vi "Relative Coordinates.vi"(1 "All Coordinates":cluster{"X":dbl, "Y":dbl}[](array[cluster]), 2 "Command Coordinates":cluster{"X":dbl, "Y":dbl}[](array[cluster])) -> (0 "Adjusted Command Coordinates":cluster{"X":dbl, "Y":dbl}[](array[cluster]))   [LabVIEW 2019]
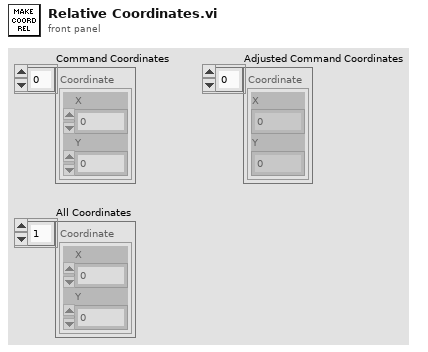
[diagram p1: front panel]
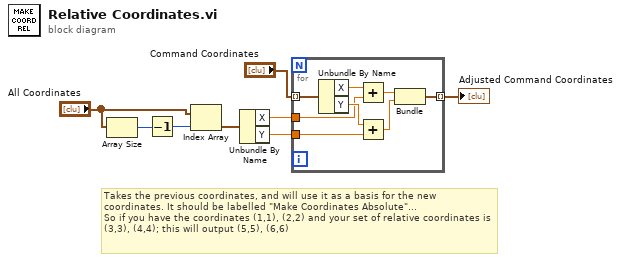
[diagram p0: block diagram]
diagram:
  # "Takes the previous coordinates, and will use it as a basis for the new coordinates. It should be labelled \"Make Coordinates Absolute\"...\nSo if you have the coordinates (1,1), (2,2) and your set of relative coordinates is (3,3), (4,4); this will output (5,5), (6,6)"
  n1 = Array Size(array="All Coordinates") -> (size(s)=w1:i32)
  n2 = Decrement(x=w1) -> (x-1=w2:i32)
  n3 = Index Array(array="All Coordinates", index=w2) -> (element=w5:cluster{"X":dbl, "Y":dbl})
  n4 = Unbundle By Name(w5) -> ("X"=w6:dbl, "Y"=w7:dbl)
  n5 = for {
    tunnel: "Command Coordinates" -> [w16] mode=indexing
    tunnel: w6 -> [w13]
    tunnel: w7 -> [w12]
    tunnel: [w9] -> w8 mode=indexing
    n6 = Unbundle By Name(w16) -> ("X"=w14:dbl, "Y"=w15:dbl)
    n7 = Add(x=w14, y=w13) -> (x+y=w11:dbl)
    n8 = Add(x=w15, y=w12) -> (x+y=w10:dbl)
    n9 = Bundle(w11, w10) -> (w9:cluster{dbl, dbl})  [unwired: 1 in]
  }
  "Adjusted Command Coordinates" <- w8
